vi "select_timezones.vi"(7 "connection_reference":T1, 8 "error in (no error)":errorcluster) -> (0 "error out":errorcluster, 3 "timezones":T2[](array[typedef]) {"utc_offset" format="%<%H:%M:%S>t"})   [LabVIEW 2015, in "lv-example-postgres.lvlib"]
uses:
  lv-example-postgres.lvlib
  _controls/timezone.ctl
  <vilib>/addons/database/Connection.llb/Conn ObjectReference.ctl
  <vilib>/addons/database/Connection.llb/Conn Execute.vi
  <vilib>/addons/database/Recordset.llb/Rec Fetch Recordset Data (R).vi
  <vilib>/addons/database/Recordset.llb/Rec Destroy - Connection.vi
  <vilib>/addons/database/NI_Database_API.lvlib
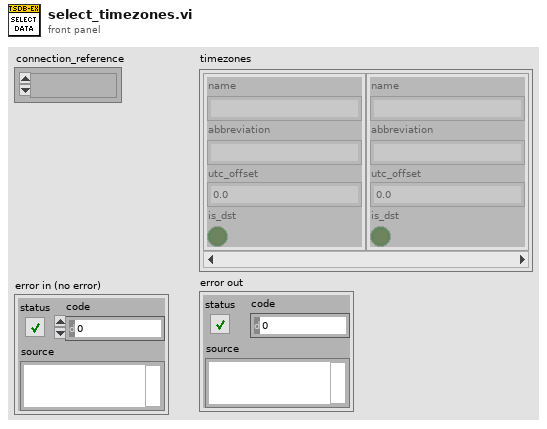
[diagram p1: front panel]
types:
  T1 = typedef "NI_Database_API.lvlib/Conn ObjectReference.ctl" = refnum<k1>
  T2 = typedef "lv-example-postgres.lvlib/timezone.ctl" = cluster{"name":string, "abbreviation":string, "utc_offset":dbl, "is_dst":bool}
  T3 = typedef "NI_Database_API.lvlib/Rec ObjectReference.ctl" = refnum<k1>
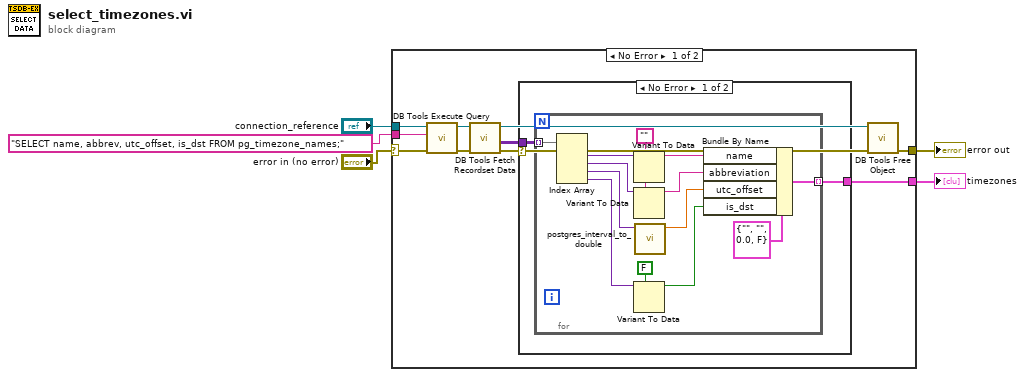
[diagram p0: block diagram]
diagram:
  n1 = case shown="No Error" "error in (no error)" {
    selector: "error in (no error)" -> [w10 w31]
    tunnel: "connection_reference" -> [w11 _]
    tunnel: [w15 w31] -> w3
    tunnel: "SELECT name, abbrev, utc_offset, is_dst FROM pg_timezone_names;" ("format string") -> [w9 _]
    tunnel: [w7 _] -> w1
    frame No Error {
      n2 = call-poly <vilib>:"DB Tools Execute Query.vi"("error in (no error)"=w10, "SQL query"=w9, "connection reference"=w11) -> ("error out"=w12:errorcluster, "recordset reference"=w14:T3)  [unwired: 5 in]
      n3 = call-poly <vilib>:"DB Tools Fetch Recordset Data.vi"("error in (no error)"=w12, "recordset reference"=w14) -> ("error out"=w6:errorcluster, "recordset data"=w8:variant[][], "recordset reference out"=w13:T3)  [unwired: 3 in]
      n4 = case shown="No Error" w6 {
        tunnel: w8 -> [w17 _]
        tunnel: [w16 _] -> w7
        frame No Error {
          n5 = for {
            tunnel: w17 -> [w30] mode=indexing
            tunnel: [w28] -> w16 mode=indexing
            w25 = ""
            n6 = Index Array(array=w30) -> (element #1=w27:variant, element #2=w26:variant, element #3=w19:variant, element #4=w20:variant)  [unwired: 4 in]
            n7 = Variant To Data(type=w25, Variant=w27) -> (data=w23:string)  [unwired: 1 in, 1 out]
            n8 = Variant To Data(type=w25, Variant=w26) -> (data=w22:string)  [unwired: 1 in, 1 out]
            n9 = Variant To Data(type=FALSE, Variant=w20) -> (data=w21:bool)  [unwired: 1 in, 1 out]
            n10 = call "postgres_interval_to_double.vi"("postgres_interval"=w19) -> ("labview_interval"=w18:dbl)  [unwired: 9 in, 1 out]
            n11 = Bundle By Name(cluster=T2 {"name"="", "abbreviation"="", "utc_offset"=0.0, "is_dst"=FALSE} ("timezone"), "name"=w23, "abbreviation"=w22, "utc_offset"=w18, "is_dst"=w21) -> (w28:T2)
          }
        }
        frame Error {
        }
      }
      n12 = call-poly <vilib>:"DB Tools Free Object.vi"("error in (no error)"=w6, "recordset reference"=w13) -> ("error out"=w15:errorcluster)  [unwired: 8 in, 1 out]
    }
    frame Error {
    }
  }
  "timezones" <- w1
  "error out" <- w3
